vi "Actor Core.vi"(8 "error in":errorcluster, 11 "Nested in":refnum<class "DataLoggerUI.lvclass">) -> (0 "error out":errorcluster, 3 "Actor out":refnum<class "Actor.lvclass">)   [LabVIEW 2020, in "DataLogger.lvlib" / "DataLoggerUI.lvclass"]
doc: "(<B>Filename</B>: Actor Framework.lvlib:Actor.lvclass:Actor Core.vi)\n\nReceives messages to the actor, reacts to them, and initiates any error handling that may shut the actor down.\n\nDescendant classes may override this VI to append parallel tasks for the actor to complete while it handles messages. Overrides use the Call Parent Method node."
uses:
  DataLoggerUI.lvclass
  <vilib>/ActorFramework/Actor/Actor.lvclass
  <vilib>/ActorFramework/Stop Msg/Stop Msg.lvclass
  Interface/DataListener Messages/OnDataChange Msg/OnDataChange Msg.lvclass
  Model/Hardware Abstraction Layer/Component/Device/Device/DataExchange.ctl
  Interface/DataListener/DataListener.lvclass
  C:/Program Files/National Instruments/LabVIEW 2020/vi.lib/ActorFramework/Actor/Actor.lvclass
  E:/Development/DevHardSoftware/MicroscopyFramework/DataLoggerUI/DataLoggerUI.lvclass
  E:/Development/DevHardSoftware/MicroscopyFramework/Interface/DataListener/DataListener.lvclass
panel:
  out "RawImage":T1(plugin-control)
  in  "File Suffix":string
  in  "Save Path":path
  in  "Alert when finish?":bool
  in  "SingleStack?":bool
  in  "StreamToDisk?":bool
  # "Save Image Mode"
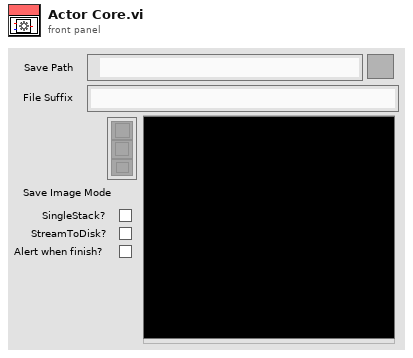
[diagram p1: front panel]
types:
  T1 = typedef "IMAQ Image.ctl" = refnum<image>
  T2 = cluster{"Stop":refnum<user-event>, "ImagePreview":refnum<user-event>}
  T3 = cluster{"StreamToDisk?":bool, "SingleStack?":bool, "Alert when finish?":bool, "TiffFileFullPath":path, "StreamFileFullPath":path}
  T4 = typedef "DataListener.lvclass/DataExchange.ctl" = cluster{"Source":string, "Destination":string, "Description":string, "value":variant}
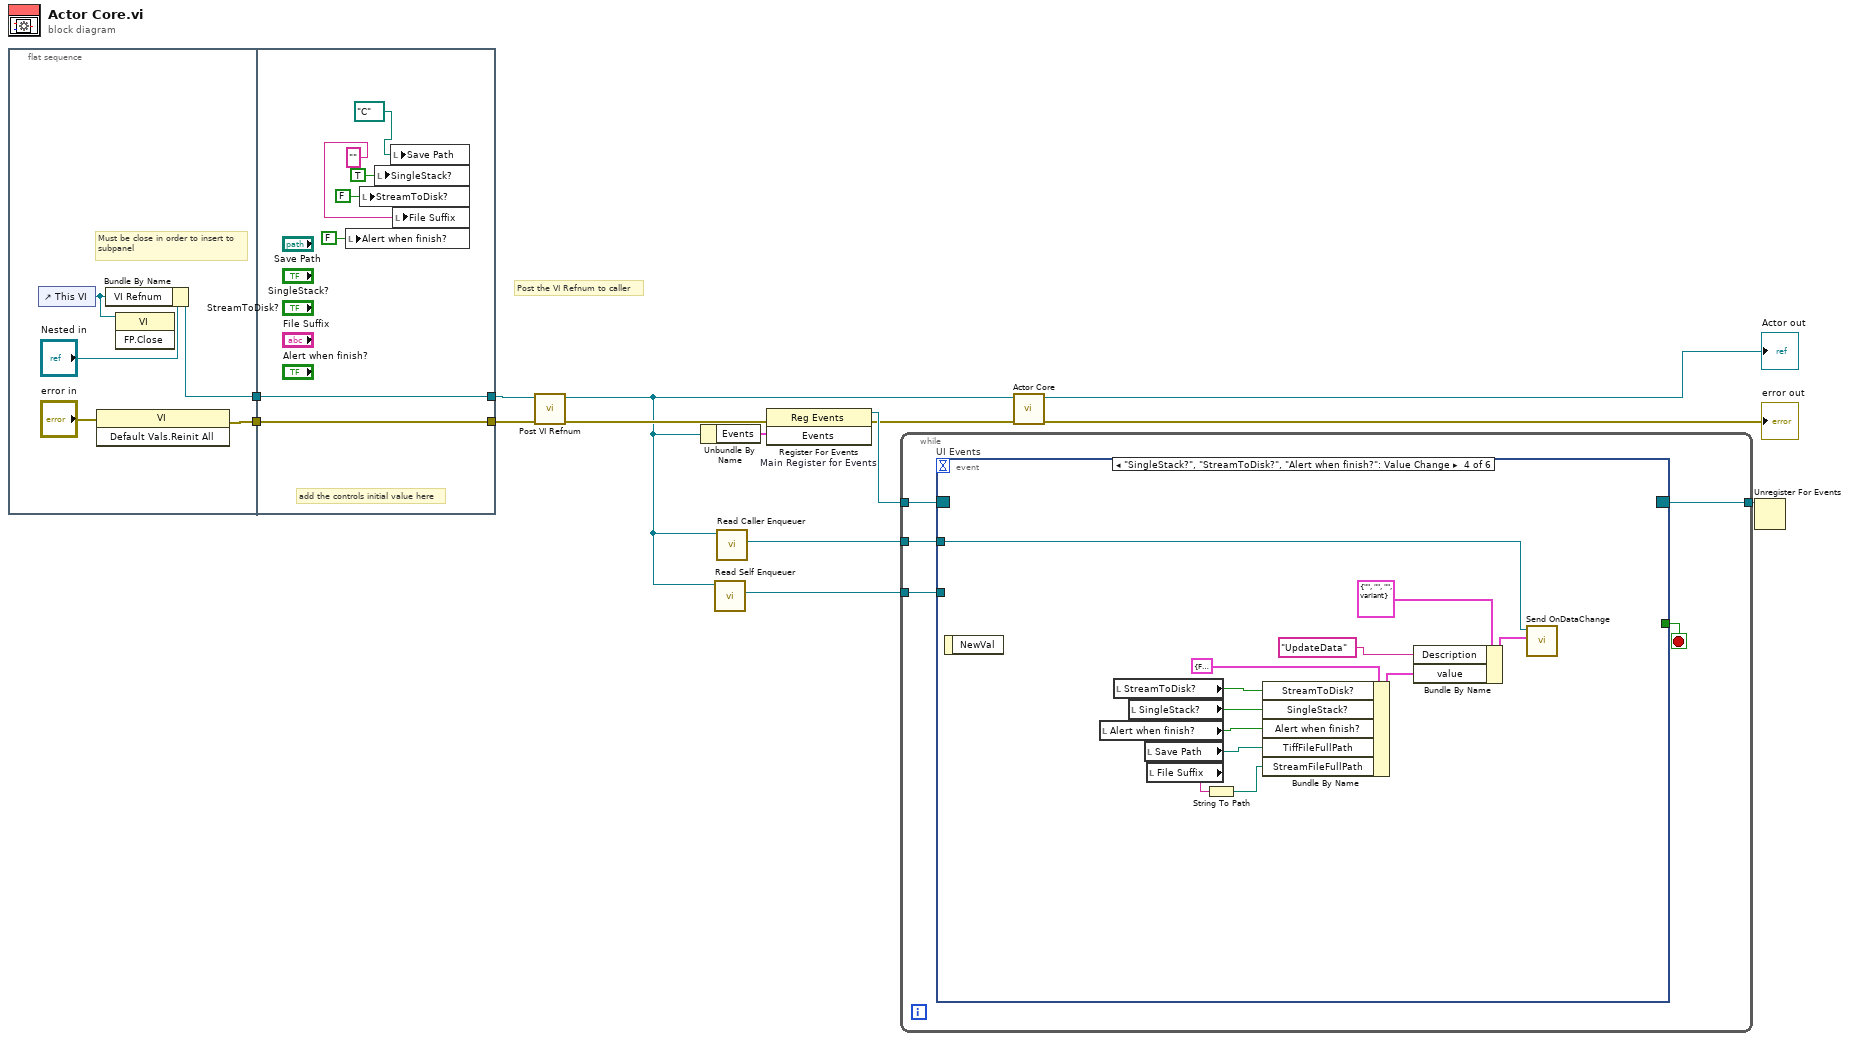
[diagram p0: block diagram]
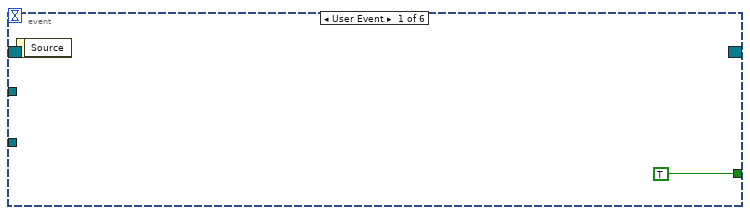
[diagram p2: hidden frame]
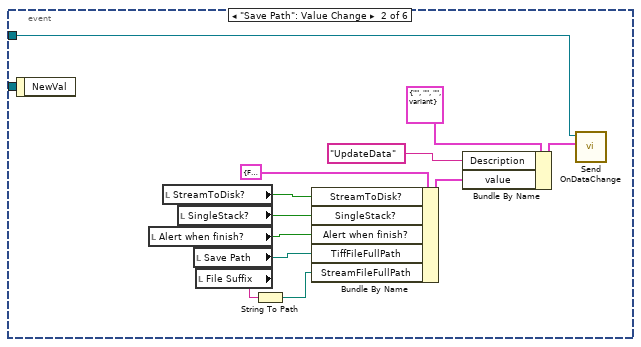
[diagram p3: hidden frame]
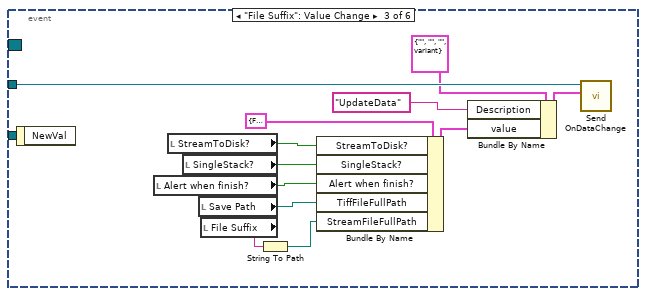
[diagram p4: hidden frame]
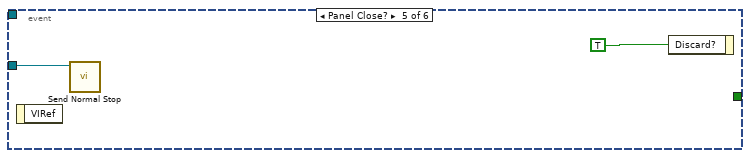
[diagram p5: hidden frame]
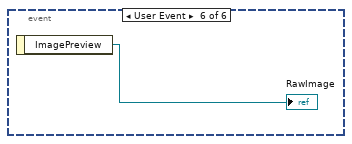
[diagram p6: hidden frame]
diagram:
  # "Post the VI Refnum to caller"
  n1 = flat-sequence {
    tunnel: [w17] -> w6
    tunnel: [w16] -> w5
    tunnel: [w25] -> w3
    tunnel: [w26] -> w7
    tunnel: w6 -> [w26]
    tunnel: w5 -> [w25]
    frame #0 {
      # "Must be close in order to insert to\nsubpanel"
      n2 = control-ref of="This VI"() -> (w15:refnum<vi>)
      n3 = invoke class="VI" method="Default Vals.Reinit All"(error in="error in") -> (error out=w17:errorcluster)  [unwired: 2 in, 2 out]
      n4 = Bundle By Name(cluster="Nested in", "VI Refnum"=w15) -> (w16:refnum<class "DataLoggerUI.lvclass">)
      n5 = invoke class="VI" method="FP.Close"(reference=w15) -> ()  [unwired: 2 in, 3 out]
    }
    frame #1 {
      # "add the controls initial value here"
      n6 = local write "Alert when finish?"(FALSE ("Alert when finish?")) -> ()
      n7 = local write "StreamToDisk?"(FALSE ("StreamToDisk?")) -> ()
      n8 = local write "SingleStack?"(TRUE ("SingleStack?")) -> ()
      n9 = local write "Save Path"(path "C:/" ("Save Path")) -> ()
      n10 = local write "File Suffix"("" ("File Suffix")) -> ()
    }
  }
  n11 = call-dynamic "Post VI Refnum.vi"("error in (no error)"=w7, "Controller Template in"=w3) -> ("error out"=w4:errorcluster, "Controller Template out"=w1:refnum<class "DataLoggerUI.lvclass">)  [unwired: 8 in]
  n12 = Unbundle By Name(w1) -> ("Events"=w11:T2)
  n13 = call <vilib>:"Read Self Enqueuer.vi"("Actor"=w1) -> ("Self Enqueuer"=w9:refnum<class "Message Enqueuer.lvclass">)  [unwired: 10 in]
  n14 = call <vilib>:"Read Caller Enqueuer.vi"("Actor"=w1) -> ("Caller Enqueuer"=w2:refnum<class "Message Enqueuer.lvclass">)  [unwired: 10 in]
  n15 = register-events "Main Register for Events"(error in=w4, w11) -> (reference out=w12:refnum<event-registration>, error out=w8:errorcluster)  [unwired: 1 in]
  n16 = while {
    tunnel: w12 -> [w31]
    tunnel: [w29] -> w10
    tunnel: w9 -> [w28]
    tunnel: w2 -> [w27]
    stop <- w30 stop-if-true
    n17 = event "UI Events" shown="[3] \"SingleStack?\", \"StreamToDisk?\", \"Alert when finish?\": Value Change" {
      selector: w31 -> [_ _ _ _ _ _]
      dyn-events: [_ _ _ _ _ _] -> w29
      timeout: _ -> [_ _ _ _ _ _]
      tunnel: [TRUE _ _ _ _ _] -> w30
      tunnel: w28 -> [_ _ _ _ w69 _]
      tunnel: w27 -> [_ w33 w56 w57 _ _]
      event User Event {
        n18 = event-data() -> ()  [unwired: 1 in, 1 out]
      }
      event "Save Path": Value Change {
        n19 = event-data() -> ()  [unwired: 1 in, 1 out]
        n20 = local read "Alert when finish?"() -> (w37:bool)
        n21 = local read "StreamToDisk?"() -> (w39:bool)
        n22 = local read "SingleStack?"() -> (w38:bool)
        n23 = local read "Save Path"() -> (w36:path)
        n24 = local read "File Suffix"() -> (w35:string)
        n25 = String To Path(string=w35) -> (path=w34:path)
        n26 = Bundle By Name(cluster=T3 {"StreamToDisk?"=FALSE, "SingleStack?"=FALSE, "Alert when finish?"=FALSE, "TiffFileFullPath"=path "", "StreamFileFullPath"=path ""} ("Images Saving"), "StreamToDisk?"=w39, "SingleStack?"=w38, "Alert when finish?"=w37, "TiffFileFullPath"=w36, "StreamFileFullPath"=w34) -> (w40:T3)
        n27 = Bundle By Name(cluster=T4 {"Source"="", "Destination"="", "Description"="", "value"=variant} ("DataExchange"), "Description"="UpdateData", "value"=w40) -> (w43:T4)
        n28 = call "Send OnDataChange.vi"("DataExchange"=w43, "Message Enqueuer"=w33) -> ()  [unwired: 8 in, 2 out]
      }
      event "File Suffix": Value Change {
        n29 = event-data() -> ()  [unwired: 1 in, 1 out]
        n30 = local read "Alert when finish?"() -> (w48:bool)
        n31 = local read "StreamToDisk?"() -> (w50:bool)
        n32 = local read "SingleStack?"() -> (w49:bool)
        n33 = local read "Save Path"() -> (w47:path)
        n34 = local read "File Suffix"() -> (w46:string)
        n35 = String To Path(string=w46) -> (path=w45:path)
        n36 = Bundle By Name(cluster=T3 {"StreamToDisk?"=FALSE, "SingleStack?"=FALSE, "Alert when finish?"=FALSE, "TiffFileFullPath"=path "", "StreamFileFullPath"=path ""} ("Images Saving"), "StreamToDisk?"=w50, "SingleStack?"=w49, "Alert when finish?"=w48, "TiffFileFullPath"=w47, "StreamFileFullPath"=w45) -> (w51:T3)
        n37 = Bundle By Name(cluster=T4 {"Source"="", "Destination"="", "Description"="", "value"=variant} ("DataExchange"), "Description"="UpdateData", "value"=w51) -> (w54:T4)
        n38 = call "Send OnDataChange.vi"("DataExchange"=w54, "Message Enqueuer"=w56) -> ()  [unwired: 8 in, 2 out]
      }
      event "SingleStack?", "StreamToDisk?", "Alert when finish?": Value Change {
        n39 = event-data() -> ()  [unwired: 1 in, 1 out]
        n40 = local read "Alert when finish?"() -> (w64:bool)
        n41 = local read "StreamToDisk?"() -> (w66:bool)
        n42 = local read "SingleStack?"() -> (w65:bool)
        n43 = local read "Save Path"() -> (w63:path)
        n44 = local read "File Suffix"() -> (w62:string)
        n45 = String To Path(string=w62) -> (path=w61:path)
        n46 = Bundle By Name(cluster=T3 {"StreamToDisk?"=FALSE, "SingleStack?"=FALSE, "Alert when finish?"=FALSE, "TiffFileFullPath"=path "", "StreamFileFullPath"=path ""} ("Images Saving"), "StreamToDisk?"=w66, "SingleStack?"=w65, "Alert when finish?"=w64, "TiffFileFullPath"=w63, "StreamFileFullPath"=w61) -> (w67:T3)
        n47 = Bundle By Name(cluster=T4 {"Source"="", "Destination"="", "Description"="", "value"=variant} ("DataExchange"), "Description"="UpdateData", "value"=w67) -> (w68:T4)
        n48 = call "Send OnDataChange.vi"("DataExchange"=w68, "Message Enqueuer"=w57) -> ()  [unwired: 8 in, 2 out]
      }
      event Panel Close? {
        n49 = event-data() -> ()  [unwired: 1 in, 1 out]
        n50 = call <vilib>:"Send Normal Stop.vi"("Message Enqueuer"=w69) -> ()  [unwired: 10 in, 1 out]
        n51 = event-data("Discard?"=TRUE) -> ()  [unwired: 1 in, 1 out]
      }
      event User Event {
        n52 = event-data() -> ("ImagePreview"=→"RawImage":T1)  [unwired: 1 in]
      }
    }
  }
  n53 = call-parent "Actor Core.vi"("error in"=w8, "Actor in"=w1) -> ("error out"=→"error out":errorcluster, "Actor out"=→"Actor out":refnum<class "Actor.lvclass">)  [unwired: 8 in]
  n54 = Unregister For Events(event registration refnum=w10) -> ()  [unwired: 1 in, 1 out]
